vi "callibrate.vi"() -> ()   [LabVIEW 2016]
uses:
  <vilib>/LabVIEW Interface for Arduino/LabVIEW Interface for Arduino.lvlib
  <vilib>/ptbypt/NI_PtbyPt.lvlib
panel:
  out "output variable":dbl
  in  "stop":bool
  out "Filtered x":dbl format="%0.2f"
  in  "input":dbl min=0.0 max=5.0
  out "x/y":dbl
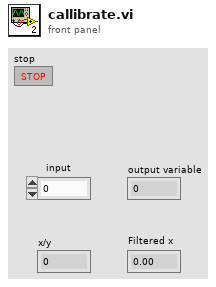
[diagram p1: front panel]
types:
  T1 = typedef "LabVIEW Interface for Arduino.lvlib/Arduino Resource.ctl" = cluster{"VISA resource":refnum<visa-resource-name>, "Board Type":T2, "Connection Type":enum8{"USB / Serial"}, "Bytes Per Packet (15)":u8}
  T2 = typedef "LabVIEW Interface for Arduino.lvlib/Board Type.ctl" = enum16{"Uno", "Dimuelanove w/Atmega 328", "Mega 2560"}
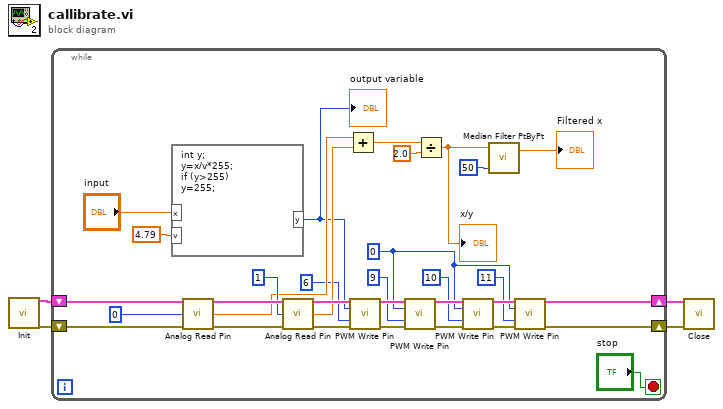
[diagram p0: block diagram]
diagram:
  n1 = call <vilib>:"Init.vi"() -> ("Arduino Resource"=w4:T1, "error out"=w2:errorcluster)  [unwired: 18 in]
  n2 = while {
    shift-right: [w12] -> w3
    shift-left: w4 -> [w36]
    shift-right: [w10] -> w1
    shift-left: w2 -> [w35]
    stop <- "stop" stop-if-true
    w9 = 0
    n3 = formula code="int y;\ny=x/v*255;\nif (y>255)\ny=255;"("x"="input", "v"=4.79 ("input variable")) -> ("y"=w7:i32)
    "output variable" <- w7
    n4 = call <vilib>:"Analog Read Pin.vi"("Arduino Resource"=w36, "Analog Input Pin (0)"=u8 0, "error in"=w35) -> ("Arduino Resource"=w33:T1, "Voltage"=w28:dbl, "error out"=w31:errorcluster)  [unwired: 10 in]
    n5 = call <vilib>:"Analog Read Pin.vi"("Arduino Resource"=w33, "Analog Input Pin (0)"=u8 1, "error in"=w31) -> ("Arduino Resource"=w32:T1, "Voltage"=w27:dbl, "error out"=w30:errorcluster)  [unwired: 10 in]
    n6 = Add(x=w28, y=w27) -> (x+y=w25:dbl)
    n7 = call <vilib>:"PWM Write Pin.vi"("Arduino Resource"=w32, "Duty Cycle (0 - 255)"=w7, "PWM Pin (3)"=u8 6, "error in"=w30) -> ("Arduino Resource"=w19:T1, "error out"=w17:errorcluster)  [unwired: 10 in]
    n8 = call <vilib>:"PWM Write Pin.vi"("Arduino Resource"=w19, "Duty Cycle (0 - 255)"=w9, "PWM Pin (3)"=u8 9, "error in"=w17) -> ("Arduino Resource"=w18:T1, "error out"=w16:errorcluster)  [unwired: 10 in]
    n9 = Divide(x=w25, y=2.0) -> (x/y=w23:dbl)
    "x/y" <- w23
    n10 = call <vilib>:"PWM Write Pin.vi"("Arduino Resource"=w18, "Duty Cycle (0 - 255)"=w9, "PWM Pin (3)"=u8 10, "error in"=w16) -> ("Arduino Resource"=w13:T1, "error out"=w11:errorcluster)  [unwired: 10 in]
    n11 = call <vilib>:"Median Filter PtByPt.vi"("rank"=50, "x"=w23) -> ("Filtered x"=→"Filtered x":dbl)  [unwired: 2 in, 1 out]
    n12 = call <vilib>:"PWM Write Pin.vi"("Arduino Resource"=w13, "Duty Cycle (0 - 255)"=w9, "PWM Pin (3)"=u8 11, "error in"=w11) -> ("Arduino Resource"=w12:T1, "error out"=w10:errorcluster)  [unwired: 10 in]
  }
  n13 = call <vilib>:"Close.vi"("Arduino Resource"=w3, "error in"=w1) -> ()  [unwired: 13 in, 1 out]
